vi "FT10_Semi-Auto 2 Activate Port.vi"(7 "Wait Time (ms)":i32, 9 "Mode in":T1, 10 "Port in":T2, 11 "Activation Method in":T4) -> (1 "Mode out":T1, 2 "Port out":T2, 3 "output cluster":T3)   [LabVIEW 2024]
uses:
  Controls/Control_Semi-Auto 2 Activation Method.ctl
  Controls/Control_Semi-Auto Port.ctl
  Controls/Control_Semi-Auto Mode.ctl
  Controls/Control_Command Cluster.ctl
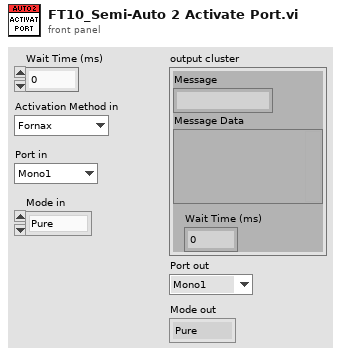
[diagram p1: front panel]
types:
  T1 = typedef "Control_Semi-Auto Mode.ctl" = enum16{"Pure", "Blend", "Spray", "Fulgerate", "Standard", "Macro", "Precision", "Ligasure", "Error"}
  T2 = typedef "Control_Semi-Auto Port.ctl" = enum16{"Mono1", "Mono2", "Bipolar", "Ligasure", "Error"}
  T3 = typedef "Control_Command Cluster.ctl" = cluster{"Message":string, "Message Data":variant, "Wait Time (ms)":i32}
  T4 = typedef "Control_Semi-Auto 2 Activation Method.ctl" = enum16{"Fornax", "Handswitch", "Footswitch"}
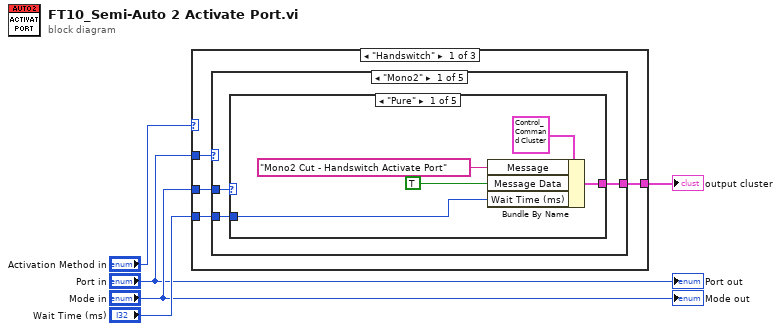
[diagram p0: block diagram]
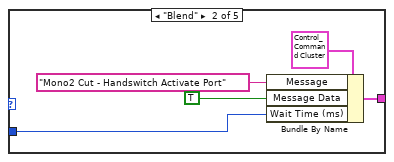
[diagram p2: hidden frame]
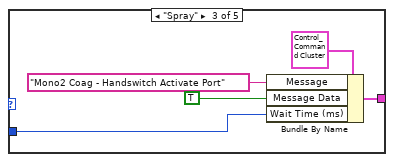
[diagram p3: hidden frame]
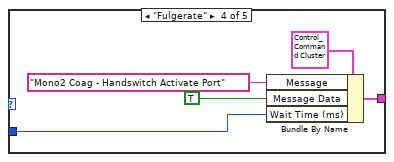
[diagram p4: hidden frame]
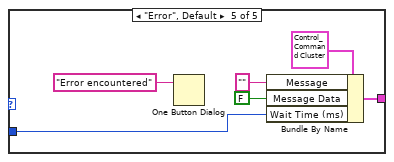
[diagram p5: hidden frame]
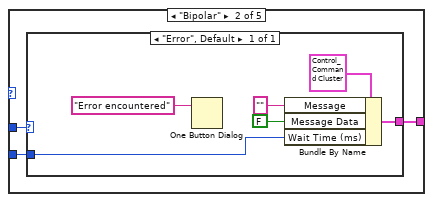
[diagram p6: hidden frame]
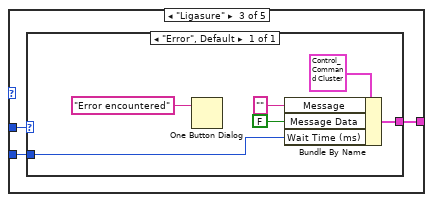
[diagram p7: hidden frame]
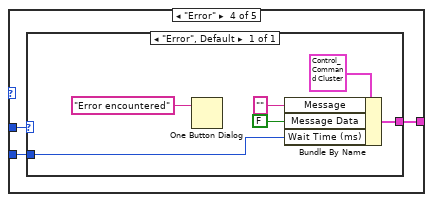
[diagram p8: hidden frame]
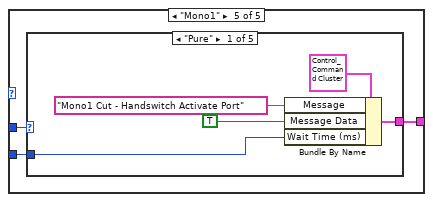
[diagram p9: hidden frame]
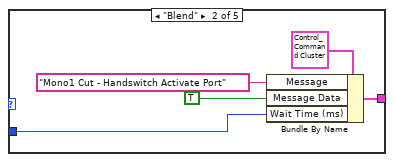
[diagram p10: hidden frame]
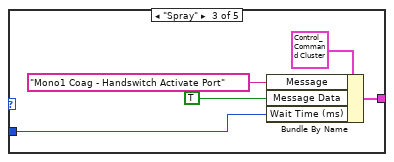
[diagram p11: hidden frame]
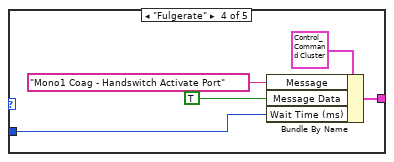
[diagram p12: hidden frame]
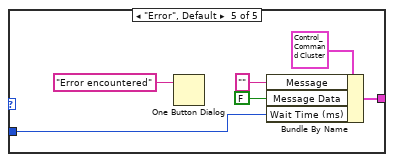
[diagram p13: hidden frame]
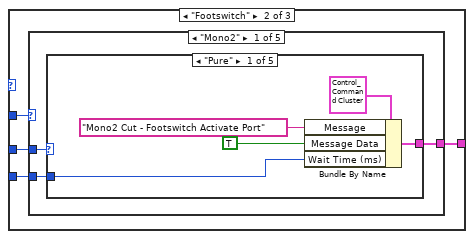
[diagram p14: hidden frame]
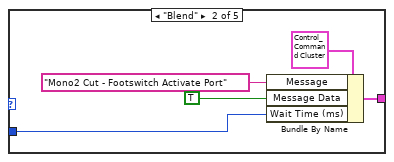
[diagram p15: hidden frame]
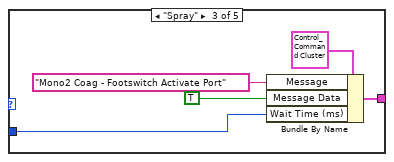
[diagram p16: hidden frame]
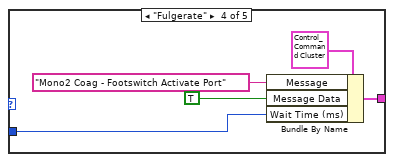
[diagram p17: hidden frame]
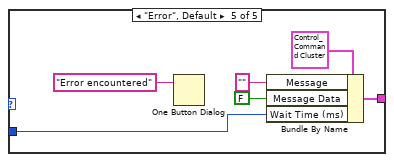
[diagram p18: hidden frame]
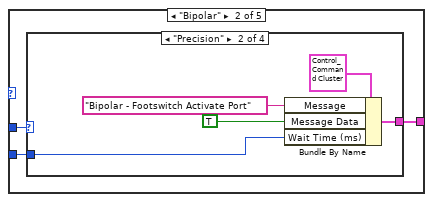
[diagram p19: hidden frame]
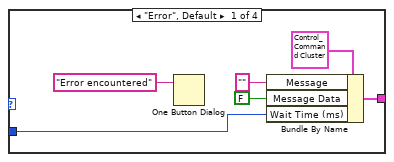
[diagram p20: hidden frame]
diagram:
  n1 = case shown="\"Handswitch\"" "Activation Method in" {
    tunnel: [w9 w98 w202] -> w1
    tunnel: "Port in" -> [w8 w97 w201]
    tunnel: "Mode in" -> [w7 w96 w200]
    tunnel: "Wait Time (ms)" -> [w6 w95 w199]
    frame "Handswitch" {
      n2 = case shown="\"Mono2\"" w8 {
        tunnel: [w12 w41 w50 w59 w68] -> w9
        tunnel: w7 -> [w11 w40 w49 w58 w67]
        tunnel: w6 -> [w10 w39 w48 w57 w66]
        frame "Mono2" {
          n3 = case shown="\"Pure\"" w11 {
            tunnel: [w16 w21 w26 w31 w37] -> w12
            tunnel: w10 -> [w13 w18 w23 w28 w34]
            frame "Pure" {
              n4 = Bundle By Name(cluster=T3 {"Message"="", "Message Data"=variant, "Wait Time (ms)"=0}, "Message"="Mono2 Cut - Handswitch Activate Port", "Message Data"=TRUE ("data"), "Wait Time (ms)"=w13) -> (w16:T3)
            }
            frame "Blend" {
              n5 = Bundle By Name(cluster=T3 {"Message"="", "Message Data"=variant, "Wait Time (ms)"=0}, "Message"="Mono2 Cut - Handswitch Activate Port", "Message Data"=TRUE ("data"), "Wait Time (ms)"=w18) -> (w21:T3)
            }
            frame "Spray" {
              n6 = Bundle By Name(cluster=T3 {"Message"="", "Message Data"=variant, "Wait Time (ms)"=0}, "Message"="Mono2 Coag - Handswitch Activate Port", "Message Data"=TRUE ("data"), "Wait Time (ms)"=w23) -> (w26:T3)
            }
            frame "Fulgerate" {
              n7 = Bundle By Name(cluster=T3 {"Message"="", "Message Data"=variant, "Wait Time (ms)"=0}, "Message"="Mono2 Coag - Handswitch Activate Port", "Message Data"=TRUE ("data"), "Wait Time (ms)"=w28) -> (w31:T3)
            }
            frame "Error", Default {
              n8 = One Button Dialog(message="Error encountered") -> ()  [unwired: 1 in, 1 out]
              n9 = Bundle By Name(cluster=T3 {"Message"="", "Message Data"=variant, "Wait Time (ms)"=0}, "Message"="", "Message Data"=FALSE ("data"), "Wait Time (ms)"=w34) -> (w37:T3)
            }
          }
        }
        frame "Bipolar" {
          n10 = case shown="\"Error\", Default" w40 {
            tunnel: [w46] -> w41
            tunnel: w39 -> [w43]
            frame "Error", Default {
              n11 = One Button Dialog(message="Error encountered") -> ()  [unwired: 1 in, 1 out]
              n12 = Bundle By Name(cluster=T3 {"Message"="", "Message Data"=variant, "Wait Time (ms)"=0}, "Message"="", "Message Data"=FALSE ("data"), "Wait Time (ms)"=w43) -> (w46:T3)
            }
          }
        }
        frame "Ligasure" {
          n13 = case shown="\"Error\", Default" w49 {
            tunnel: [w55] -> w50
            tunnel: w48 -> [w52]
            frame "Error", Default {
              n14 = One Button Dialog(message="Error encountered") -> ()  [unwired: 1 in, 1 out]
              n15 = Bundle By Name(cluster=T3 {"Message"="", "Message Data"=variant, "Wait Time (ms)"=0}, "Message"="", "Message Data"=FALSE ("data"), "Wait Time (ms)"=w52) -> (w55:T3)
            }
          }
        }
        frame "Error" {
          n16 = case shown="\"Error\", Default" w58 {
            tunnel: [w64] -> w59
            tunnel: w57 -> [w61]
            frame "Error", Default {
              n17 = One Button Dialog(message="Error encountered") -> ()  [unwired: 1 in, 1 out]
              n18 = Bundle By Name(cluster=T3 {"Message"="", "Message Data"=variant, "Wait Time (ms)"=0}, "Message"="", "Message Data"=FALSE ("data"), "Wait Time (ms)"=w61) -> (w64:T3)
            }
          }
        }
        frame "Mono1" {
          n19 = case shown="\"Pure\"" w67 {
            tunnel: [w72 w77 w82 w87 w93] -> w68
            tunnel: w66 -> [w69 w74 w79 w84 w90]
            frame "Pure" {
              n20 = Bundle By Name(cluster=T3 {"Message"="", "Message Data"=variant, "Wait Time (ms)"=0}, "Message"="Mono1 Cut - Handswitch Activate Port", "Message Data"=TRUE ("data"), "Wait Time (ms)"=w69) -> (w72:T3)
            }
            frame "Blend" {
              n21 = Bundle By Name(cluster=T3 {"Message"="", "Message Data"=variant, "Wait Time (ms)"=0}, "Message"="Mono1 Cut - Handswitch Activate Port", "Message Data"=TRUE ("data"), "Wait Time (ms)"=w74) -> (w77:T3)
            }
            frame "Spray" {
              n22 = Bundle By Name(cluster=T3 {"Message"="", "Message Data"=variant, "Wait Time (ms)"=0}, "Message"="Mono1 Coag - Handswitch Activate Port", "Message Data"=TRUE ("data"), "Wait Time (ms)"=w79) -> (w82:T3)
            }
            frame "Fulgerate" {
              n23 = Bundle By Name(cluster=T3 {"Message"="", "Message Data"=variant, "Wait Time (ms)"=0}, "Message"="Mono1 Coag - Handswitch Activate Port", "Message Data"=TRUE ("data"), "Wait Time (ms)"=w84) -> (w87:T3)
            }
            frame "Error", Default {
              n24 = One Button Dialog(message="Error encountered") -> ()  [unwired: 1 in, 1 out]
              n25 = Bundle By Name(cluster=T3 {"Message"="", "Message Data"=variant, "Wait Time (ms)"=0}, "Message"="", "Message Data"=FALSE ("data"), "Wait Time (ms)"=w90) -> (w93:T3)
            }
          }
        }
      }
    }
    frame "Footswitch" {
      n26 = case shown="\"Mono2\"" w97 {
        tunnel: [w101 w130 w154 w163 w172] -> w98
        tunnel: w96 -> [w100 w129 w153 w162 w171]
        tunnel: w95 -> [w99 w128 w152 w161 w170]
        frame "Mono2" {
          n27 = case shown="\"Pure\"" w100 {
            tunnel: [w105 w110 w115 w120 w126] -> w101
            tunnel: w99 -> [w102 w107 w112 w117 w123]
            frame "Pure" {
              n28 = Bundle By Name(cluster=T3 {"Message"="", "Message Data"=variant, "Wait Time (ms)"=0}, "Message"="Mono2 Cut - Footswitch Activate Port", "Message Data"=TRUE ("data"), "Wait Time (ms)"=w102) -> (w105:T3)
            }
            frame "Blend" {
              n29 = Bundle By Name(cluster=T3 {"Message"="", "Message Data"=variant, "Wait Time (ms)"=0}, "Message"="Mono2 Cut - Footswitch Activate Port", "Message Data"=TRUE ("data"), "Wait Time (ms)"=w107) -> (w110:T3)
            }
            frame "Spray" {
              n30 = Bundle By Name(cluster=T3 {"Message"="", "Message Data"=variant, "Wait Time (ms)"=0}, "Message"="Mono2 Coag - Footswitch Activate Port", "Message Data"=TRUE ("data"), "Wait Time (ms)"=w112) -> (w115:T3)
            }
            frame "Fulgerate" {
              n31 = Bundle By Name(cluster=T3 {"Message"="", "Message Data"=variant, "Wait Time (ms)"=0}, "Message"="Mono2 Coag - Footswitch Activate Port", "Message Data"=TRUE ("data"), "Wait Time (ms)"=w117) -> (w120:T3)
            }
            frame "Error", Default {
              n32 = One Button Dialog(message="Error encountered") -> ()  [unwired: 1 in, 1 out]
              n33 = Bundle By Name(cluster=T3 {"Message"="", "Message Data"=variant, "Wait Time (ms)"=0}, "Message"="", "Message Data"=FALSE ("data"), "Wait Time (ms)"=w123) -> (w126:T3)
            }
          }
        }
        frame "Bipolar" {
          n34 = case shown="\"Precision\"" w129 {
            tunnel: [w135 w140 w145 w150] -> w130
            tunnel: w128 -> [w132 w139 w144 w149]
            frame "Error", Default {
              n35 = One Button Dialog(message="Error encountered") -> ()  [unwired: 1 in, 1 out]
              n36 = Bundle By Name(cluster=T3 {"Message"="", "Message Data"=variant, "Wait Time (ms)"=0}, "Message"="", "Message Data"=FALSE ("data"), "Wait Time (ms)"=w132) -> (w135:T3)
            }
            frame "Precision" {
              n37 = Bundle By Name(cluster=T3 {"Message"="", "Message Data"=variant, "Wait Time (ms)"=0}, "Message"="Bipolar - Footswitch Activate Port", "Message Data"=TRUE ("data"), "Wait Time (ms)"=w139) -> (w140:T3)
            }
            frame "Macro" {
              n38 = Bundle By Name(cluster=T3 {"Message"="", "Message Data"=variant, "Wait Time (ms)"=0}, "Message"="Bipolar - Footswitch Activate Port", "Message Data"=TRUE ("data"), "Wait Time (ms)"=w144) -> (w145:T3)
            }
            frame "Standard" {
              n39 = Bundle By Name(cluster=T3 {"Message"="", "Message Data"=variant, "Wait Time (ms)"=0}, "Message"="Bipolar - Footswitch Activate Port", "Message Data"=TRUE ("data"), "Wait Time (ms)"=w149) -> (w150:T3)
            }
          }
        }
        frame "Ligasure" {
          n40 = case shown="\"Error\", Default" w153 {
            tunnel: [w159] -> w154
            tunnel: w152 -> [w156]
            frame "Error", Default {
              n41 = One Button Dialog(message="Error encountered") -> ()  [unwired: 1 in, 1 out]
              n42 = Bundle By Name(cluster=T3 {"Message"="", "Message Data"=variant, "Wait Time (ms)"=0}, "Message"="", "Message Data"=FALSE ("data"), "Wait Time (ms)"=w156) -> (w159:T3)
            }
          }
        }
        frame "Error" {
          n43 = case shown="\"Error\", Default" w162 {
            tunnel: [w168] -> w163
            tunnel: w161 -> [w165]
            frame "Error", Default {
              n44 = One Button Dialog(message="Error encountered") -> ()  [unwired: 1 in, 1 out]
              n45 = Bundle By Name(cluster=T3 {"Message"="", "Message Data"=variant, "Wait Time (ms)"=0}, "Message"="", "Message Data"=FALSE ("data"), "Wait Time (ms)"=w165) -> (w168:T3)
            }
          }
        }
        frame "Mono1" {
          n46 = case shown="\"Pure\"" w171 {
            tunnel: [w176 w181 w186 w191 w197] -> w172
            tunnel: w170 -> [w173 w178 w183 w188 w194]
            frame "Pure" {
              n47 = Bundle By Name(cluster=T3 {"Message"="", "Message Data"=variant, "Wait Time (ms)"=0}, "Message"="Mono1 Cut - Footswitch Activate Port", "Message Data"=TRUE ("data"), "Wait Time (ms)"=w173) -> (w176:T3)
            }
            frame "Blend" {
              n48 = Bundle By Name(cluster=T3 {"Message"="", "Message Data"=variant, "Wait Time (ms)"=0}, "Message"="Mono1 Cut - Footswitch Activate Port", "Message Data"=TRUE ("data"), "Wait Time (ms)"=w178) -> (w181:T3)
            }
            frame "Spray" {
              n49 = Bundle By Name(cluster=T3 {"Message"="", "Message Data"=variant, "Wait Time (ms)"=0}, "Message"="Mono1 Coag - Footswitch Activate Port", "Message Data"=TRUE ("data"), "Wait Time (ms)"=w183) -> (w186:T3)
            }
            frame "Fulgerate" {
              n50 = Bundle By Name(cluster=T3 {"Message"="", "Message Data"=variant, "Wait Time (ms)"=0}, "Message"="Mono1 Coag - Footswitch Activate Port", "Message Data"=TRUE ("data"), "Wait Time (ms)"=w188) -> (w191:T3)
            }
            frame "Error", Default {
              n51 = One Button Dialog(message="Error encountered") -> ()  [unwired: 1 in, 1 out]
              n52 = Bundle By Name(cluster=T3 {"Message"="", "Message Data"=variant, "Wait Time (ms)"=0}, "Message"="", "Message Data"=FALSE ("data"), "Wait Time (ms)"=w194) -> (w197:T3)
            }
          }
        }
      }
    }
    frame "Fornax" {
      n53 = case shown="\"Error\", Default" w201 {
        tunnel: [w205] -> w202
        tunnel: w200 -> [w204]
        tunnel: w199 -> [w203]
        frame "Error", Default {
          n54 = case shown="\"Error\", Default" w204 {
            tunnel: [w210] -> w205
            tunnel: w203 -> [w207]
            frame "Error", Default {
              n55 = One Button Dialog(message="Error encountered") -> ()  [unwired: 1 in, 1 out]
              n56 = Bundle By Name(cluster=T3 {"Message"="", "Message Data"=variant, "Wait Time (ms)"=0}, "Message"="", "Message Data"=FALSE ("data"), "Wait Time (ms)"=w207) -> (w210:T3)
            }
          }
        }
      }
    }
  }
  "output cluster" <- w1
  "Port out" <- "Port in"
  "Mode out" <- "Mode in"
